vi "Low tank level handler.vi"() -> (3 "Enum":T1)   [LabVIEW 2020]
uses:
  Estados.ctl
  Variables Globales.vi
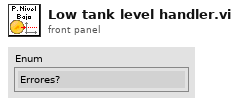
[diagram p1: front panel]
types:
  T1 = typedef "Estados.ctl" = enum16{"Errores?", "Control de válvula alt.", "Control de válvula", "Nivel bajo?", "Query nivel del tanque", "Query peso del pote", "Ajuste?", "Llenado?", "Emergencia?", "Init", "Ajuste", "Nivel Bajo", "Llenado", "Error", "Emergencia"}
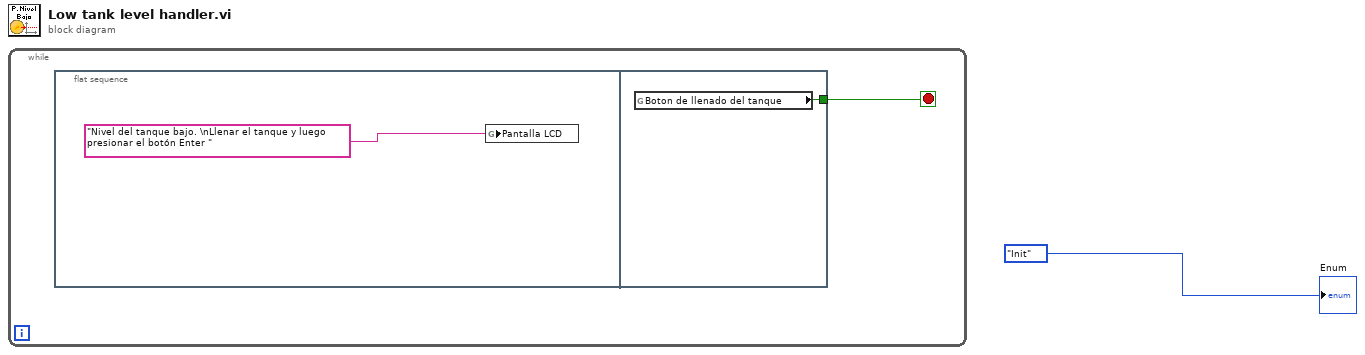
[diagram p0: block diagram]
diagram:
  n1 = while {
    stop <- w2 stop-if-true
    n2 = flat-sequence {
      tunnel: [w4] -> w2
      frame #0 {
        n3 = global write "Variables Globales.vi" "Pantalla LCD"("Nivel del tanque bajo. \nLlenar el tanque y luego presionar el botón Enter " ("string")) -> ()
      }
      frame #1 {
        n4 = global read "Variables Globales.vi" "Boton de llenado del tanque"() -> (w4:bool)
      }
    }
  }
  "Enum" <- Estados."Init"
